vi "cRIOBackplaneInfo.vi"(8 "error in (no error)":errorcluster, 11 "session in":refnum<k21>="localhost") -> (0 "error out":errorcluster, 1 "Number of Slots":i32[](array[numeric]), 2 "Chasses Info":T1[](array[typedef]))   [LabVIEW 2017, in "cRIODetectHW.lvlib"]
doc: "Gets information about the chassis used in the specified session, such as model name, model code, and serial number."
uses:
  <vilib>/addons/cRIODetectHW/cRIODetectHW.lvlib
  <vilib>/addons/cRIODetectHW/control/cRIO Product Info.ctl
  <vilib>/nisyscfg/Initialize (Control).vi
  <vilib>/nisyscfg/Find Hardware.vi
  <vilib>/nisyscfg/Close (Hardware).vi
  <vilib>/nisyscfg/Close (Filter).vi
  <resource>/objmgr/nicontrollersysapi.rc
  <resource>/objmgr/niflexrioatomicsae.rc
  <vilib>/nisyscfg/nisyscfg.lvlib
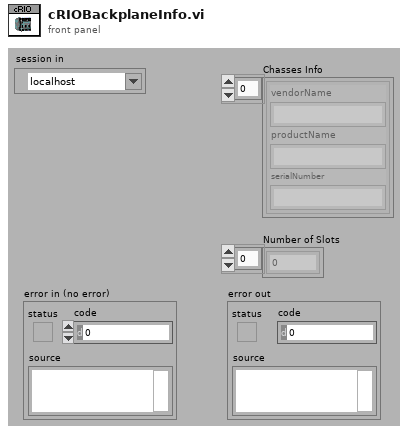
[diagram p1: front panel]
types:
  T1 = typedef "cRIODetectHW.lvlib/cRIO Product Info.ctl" = cluster{"vendorName":string, "productName":string, "serialNumber":string}
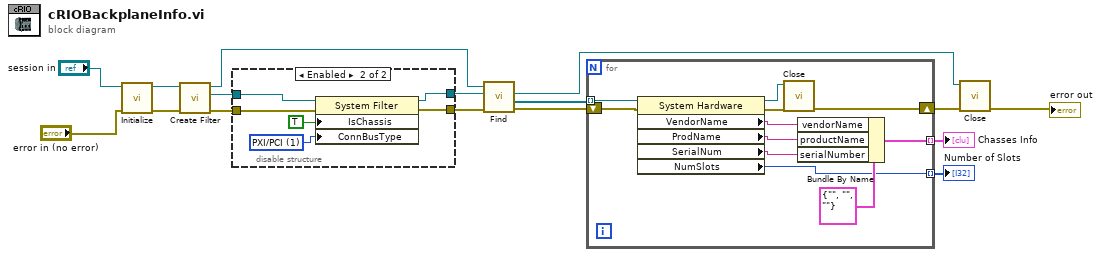
[diagram p0: block diagram]
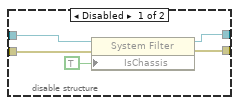
[diagram p2: hidden frame]
diagram:
  n1 = call-poly <vilib>:"Initialize.vi"("error in (no error)"="error in (no error)", "Target (localhost)"="session in") -> ("error out"=w5:errorcluster, "Session out"=w6:refnum<k21>)  [unwired: 7 in, 1 out]
  n2 = call <vilib>:"Create Filter.vi"("error in (no error)"=w5, "Session in"=w6) -> ("error out"=w15:errorcluster, "Filter out"=w16:refnum<k20>, "Session out"=w1:refnum<k21>)  [unwired: 7 in]
  n3 = disable-structure shown="Enabled" {
    disable-tunnel: w16 -> [w21 w27]
    disable-tunnel: w15 -> [w20 w26]
    disable-tunnel: [w18 w24] -> w14
    disable-tunnel: [w17 w23] -> w13
    frame Disabled {
      n4 = property class="System Filter"(reference=w21, error in=w20, "IsChassis"=TRUE ("Is Chassis")) -> (reference out=w18:refnum<k20>, error out=w17:errorcluster)
    }
    frame Enabled {
      w22 = u32 1 items=["BuiltIn/System", "PXI/PCI", "USB", "GPIB", "VXI", "Serial", "TCP/IP", "cRIO", "SCXI", "cDAQ", "SwitchBlock", "SCC", "FireWire", "Accessory", "CAN", "SwitchBlock Device"] ("Devices & Chassis:Connects To Bus Type")
      n5 = property class="System Filter"(reference=w27, error in=w26, "IsChassis"=TRUE ("Is Chassis"), "ConnBusType"=w22) -> (reference out=w24:refnum<k20>, error out=w23:errorcluster)
    }
  }
  n6 = call-poly <vilib>:"Find.vi"("error in (no error)"=w13, "Filter in"=w14, "Session in"=w1) -> ("error out"=w12:errorcluster, "Resources out"=w11:refnum<k20>[], "Filter out"=w9:refnum<k20>)  [unwired: 5 in, 1 out]
  n7 = for {
    tunnel: w11 -> [w38] mode=indexing
    shift-right: [w35] -> w10
    shift-left: w12 -> [w34]
    tunnel: [w31] -> w4 mode=indexing
    tunnel: [w28] -> w2 mode=indexing
    n8 = property class="System Hardware"(reference=w38, error in=w34) -> (reference out=w36:refnum<k20>, error out=w37:errorcluster, "VendorName"=w33:string, "ProdName"=w30:string, "SerialNum"=w29:string, "NumSlots"=w28:i32)
    n9 = call-poly <vilib>:"Close.vi"("error in (no error)"=w37, "Resource in"=w36) -> ("error out"=w35:errorcluster)  [unwired: 9 in]
    n10 = Bundle By Name(cluster=T1 {"vendorName"="", "productName"="", "serialNumber"=""} ("cRIO Backplane Info"), "vendorName"=w33, "productName"=w30, "serialNumber"=w29) -> (w31:T1)
  }
  "Chasses Info" <- w4
  "Number of Slots" <- w2
  n11 = call-poly <vilib>:"Close.vi"("error in (no error)"=w10, "Filter in"=w9) -> ("error out"=→"error out":errorcluster)  [unwired: 9 in]
